vi "Number to Match.vi"() -> ()   [LabVIEW 2023]
panel:
  out ">250":bool
  out "170 - 250":bool
  out "120-170":bool
  out "90 -120":bool
  out "65-90":bool
  out "40-65":bool
  out "20-40":bool
  out "<20":bool
  in  "Go":bool
  in  "Stop":bool
  out "Iteration Count":i32
  in  "Number to Match\nBetween 0 & 100":i16
  # "SCORE"
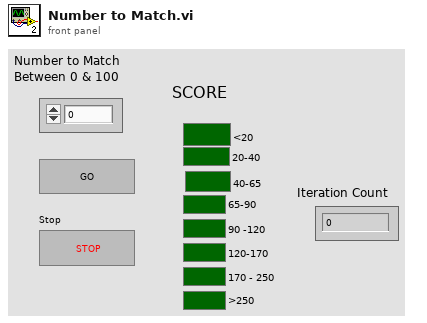
[diagram p1: front panel]
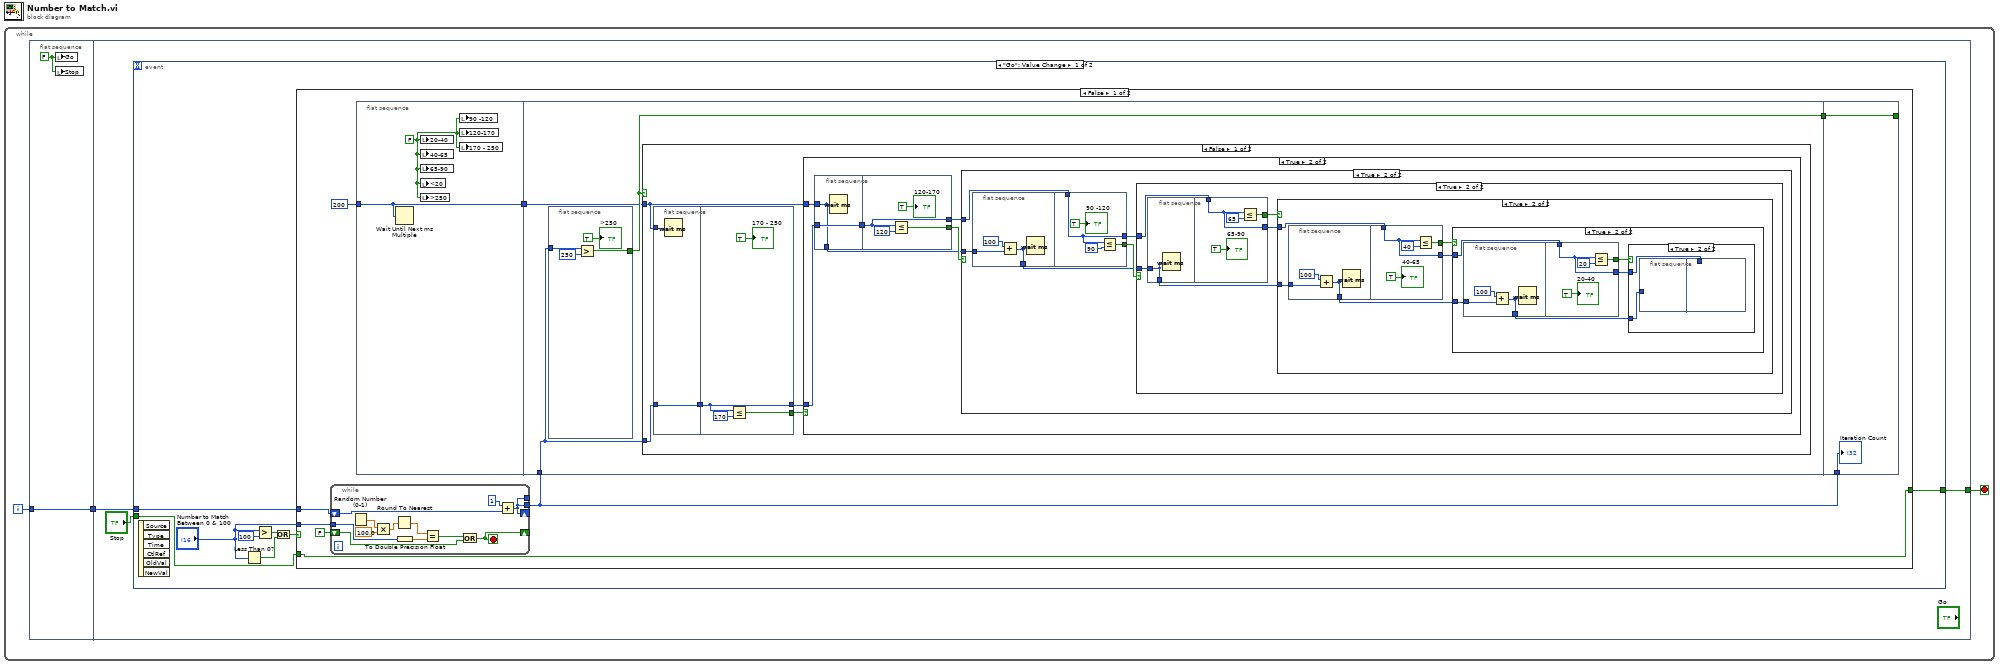
[diagram p0: block diagram]
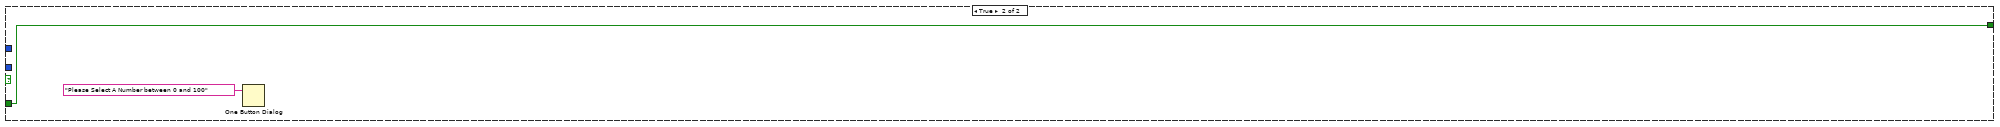
[diagram p9: hidden frame]
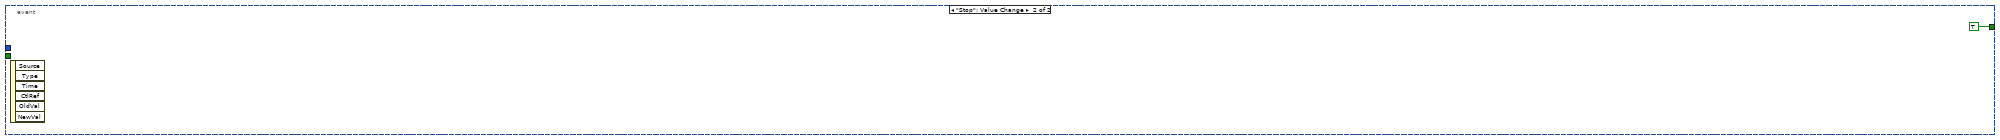
[diagram p10: hidden frame]
diagram:
  n1 = while {
    i -> [w2]
    stop <- w3 stop-if-true
    n2 = flat-sequence {
      tunnel: w2 -> [w5]
      tunnel: [w5] -> w1
      tunnel: [w8] -> w3
      tunnel: w1 -> [w7]
      frame #0 {
        w4 = FALSE ("Stop")
        n3 = local write "Go"(w4) -> ()
        n4 = local write "Stop"(w4) -> ()
      }
      frame #1 {
        n5 = event shown="[0] \"Go\": Value Change" {
          selector: _ -> [_ _]
          dyn-events: _ -> [_ _]
          timeout: _ -> [_ _]
          tunnel: [w16 TRUE ("Stop")] -> w8
          tunnel: w7 -> [w15 _]
          tunnel: "Stop" -> [w14 _]
          event "Go": Value Change {
            n6 = event-data() -> ()  [unwired: 1 in, 6 out]
            n7 = Less Than 0?(x="Number to Match\nBetween 0 & 100") -> (x < 0?=w10:bool)
            n8 = Greater?(x="Number to Match\nBetween 0 & 100", y=i16 100) -> (0:w11:bool)
            n9 = Or(x=w11, y=w10) -> (x .or. y?=w9:bool)
            n10 = case shown="False" w9 {
              tunnel: [w23 w122] -> w16
              tunnel: w15 -> [w24 _]
              tunnel: w14 -> [w23 w122]
              tunnel: "Number to Match\nBetween 0 & 100" -> [w21 _]
              frame False {
                n11 = while {
                  shift-right: [w111] -> _
                  shift-left: FALSE -> [w112]
                  shift-right: [w109] -> _
                  shift-left: w24 -> [w114]
                  tunnel: w21 -> [w110]
                  tunnel: [w109] -> _
                  tunnel: [w109] -> w18
                  stop <- w111 stop-if-true
                  n12 = Random Number (0-1)() -> (number: 0 to 1=w120:dbl)
                  n13 = Multiply(x=w120, y=100.0) -> (x*y=w118:dbl)
                  n14 = Round To Nearest(number=w118) -> (nearest integer value=w116:dbl)
                  n15 = To Double Precision Float(number=w110) -> (double precision float=w113:dbl)
                  n16 = Equal?(x=w116, y=w113) -> (x = y?=w117:bool)
                  n17 = Or(x=w117, y=w112) -> (x .or. y?=w111:bool)
                  n18 = Add(x=1, y=w114) -> (x+y=w109:i32)
                }
                n19 = flat-sequence {
                  tunnel: u32 200 ("millisecond multiple") -> [w25]
                  tunnel: [w25] -> w17
                  tunnel: w18 -> [w27]
                  tunnel: [w29] -> w19
                  tunnel: w17 -> [w28]
                  tunnel: [w108] -> _
                  tunnel: w19 -> [w108]
                  tunnel: w18 -> [w107]
                  frame #0 {
                    w26 = FALSE ("120-170")
                    n20 = Wait Until Next ms Multiple(millisecond multiple=w25) -> ()  [unwired: 1 out]
                    n21 = local write "20-40"(w26) -> ()
                    n22 = local write "40-65"(w26) -> ()
                    n23 = local write "65-90"(w26) -> ()
                    n24 = local write "<20"(w26) -> ()
                    n25 = local write ">250"(w26) -> ()
                    n26 = local write "90 -120"(w26) -> ()
                    n27 = local write "120-170"(w26) -> ()
                    n28 = local write "170 - 250"(w26) -> ()
                  }
                  frame #1 {
                    n29 = flat-sequence {
                      tunnel: [w32] -> w29
                      tunnel: w27 -> [w31]
                      frame #0 {
                        n30 = Greater?(x=w31, y=250) -> (0:w32:bool)
                        ">250" <- TRUE (">250")
                      }
                    }
                    n31 = case shown="False" w29 {
                      tunnel: w28 -> [w37 _]
                      tunnel: w27 -> [w38 _]
                      frame False {
                        n32 = flat-sequence {
                          tunnel: w38 -> [w39]
                          tunnel: w37 -> [w40]
                          tunnel: [w39] -> w36
                          tunnel: w36 -> [w42]
                          tunnel: [w43] -> w35
                          tunnel: [w42] -> w34
                          frame #0 {
                            n33 = Wait (ms)(milliseconds to wait=w40) -> ()  [unwired: 1 out]
                          }
                          frame #1 {
                            n34 = Less Or Equal?(x=w42, y=170) -> (x <= y?=w43:bool)
                            "170 - 250" <- TRUE ("170 - 250")
                          }
                        }
                        n35 = case shown="True" w35 {
                          tunnel: w37 -> [_ w48]
                          tunnel: w34 -> [_ w49]
                          frame False {
                          }
                          frame True {
                            n36 = flat-sequence {
                              tunnel: w49 -> [w102]
                              tunnel: w48 -> [w101]
                              tunnel: [w102] -> w50
                              tunnel: [w101] -> w45
                              tunnel: w50 -> [w103]
                              tunnel: [w105] -> w47
                              tunnel: [w103] -> w46
                              frame #0 {
                                n37 = Wait (ms)(milliseconds to wait=w101) -> ()  [unwired: 1 out]
                              }
                              frame #1 {
                                n38 = Less Or Equal?(x=w103, y=120) -> (x <= y?=w105:bool)
                                "120-170" <- TRUE ("170 - 250")
                              }
                            }
                            n39 = case shown="True" w47 {
                              tunnel: w46 -> [_ w55]
                              tunnel: w45 -> [_ w54]
                              frame False {
                              }
                              frame True {
                                n40 = flat-sequence {
                                tunnel: w54 -> [w95]
                                tunnel: [w94] -> w51
                                tunnel: [w99] -> w53
                                tunnel: w55 -> [w98]
                                tunnel: [w98] -> w52
                                frame #0 {
                                n41 = Add(x=u32 100, y=w95) -> (x+y=w94:u32)
                                n42 = Wait (ms)(milliseconds to wait=w94) -> ()  [unwired: 1 out]
                                }
                                frame #1 {
                                n43 = Less Or Equal?(x=w98, y=90) -> (x <= y?=w99:bool)
                                "90 -120" <- TRUE ("170 - 250")
                                }
                                }
                                n44 = case shown="True" w53 {
                                tunnel: w51 -> [_ w60]
                                tunnel: w52 -> [_ w59]
                                frame False {
                                }
                                frame True {
                                n45 = flat-sequence {
                                tunnel: w60 -> [w89]
                                tunnel: [w89] -> w57
                                tunnel: [w92] -> w58
                                tunnel: w59 -> [w90]
                                tunnel: [w90] -> w56
                                frame #0 {
                                n46 = Wait (ms)(milliseconds to wait=w89) -> ()  [unwired: 1 out]
                                }
                                frame #1 {
                                n47 = Less Or Equal?(x=w90, y=65) -> (x <= y?=w92:bool)
                                "65-90" <- TRUE ("170 - 250")
                                }
                                }
                                n48 = case shown="True" w58 {
                                tunnel: w57 -> [_ w65]
                                tunnel: w56 -> [_ w64]
                                frame False {
                                }
                                frame True {
                                n49 = flat-sequence {
                                tunnel: w65 -> [w84]
                                tunnel: [w82] -> w62
                                tunnel: [w87] -> w61
                                tunnel: w64 -> [w85]
                                tunnel: [w85] -> w63
                                frame #0 {
                                n50 = Add(x=u32 100, y=w84) -> (x+y=w82:u32)
                                n51 = Wait (ms)(milliseconds to wait=w82) -> ()  [unwired: 1 out]
                                }
                                frame #1 {
                                n52 = Less Or Equal?(x=w85, y=40) -> (x <= y?=w87:bool)
                                "40-65" <- TRUE ("170 - 250")
                                }
                                }
                                n53 = case shown="True" w61 {
                                tunnel: w63 -> [_ w70]
                                tunnel: w62 -> [_ w69]
                                frame False {
                                }
                                frame True {
                                n54 = flat-sequence {
                                tunnel: w69 -> [w76]
                                tunnel: [w75] -> w67
                                tunnel: [w80] -> w66
                                tunnel: w70 -> [w78]
                                tunnel: [w78] -> w68
                                frame #0 {
                                n55 = Add(x=u32 100, y=w76) -> (x+y=w75:u32)
                                n56 = Wait (ms)(milliseconds to wait=w75) -> ()  [unwired: 1 out]
                                }
                                frame #1 {
                                n57 = Less Or Equal?(x=w78, y=20) -> (x <= y?=w80:bool)
                                "20-40" <- TRUE ("170 - 250")
                                }
                                }
                                n58 = case shown="True" w66 {
                                tunnel: w68 -> [_ w72]
                                tunnel: w67 -> [_ w71]
                                frame False {
                                }
                                frame True {
                                n59 = flat-sequence {
                                tunnel: w71 -> [w73]
                                tunnel: w72 -> [_]
                                frame #0 {
                                n60 = Wait (ms)(milliseconds to wait=w73) -> ()  [unwired: 1 out]
                                }
                                frame #1 {
                                "<20" <- TRUE ("170 - 250")
                                }
                                }
                                }
                                }
                                }
                                }
                                }
                                }
                                }
                                }
                              }
                            }
                          }
                        }
                      }
                      frame True {
                      }
                    }
                  }
                  frame #2 {
                    "Iteration Count" <- w107
                  }
                }
              }
              frame True {
                n61 = One Button Dialog(message="Please Select A Number between 0 and 100") -> ()  [unwired: 1 in, 1 out]
              }
            }
          }
          event "Stop": Value Change {
            n62 = event-data() -> ()  [unwired: 1 in, 6 out]
          }
        }
      }
    }
  }
